vi "Global-IP_UI.vi"() -> ()   [LabVIEW 2021]
uses:
  IP_Cellular Tech Type def.ctl
  IP_Network_Type def.ctl
  IP_Type-Tydedef.ctl
panel:
  in  "IP_UI":T4(array[cluster])
  in  "IP_UI_Boolean":bool[](array[boolean])=[FALSE, FALSE, FALSE]
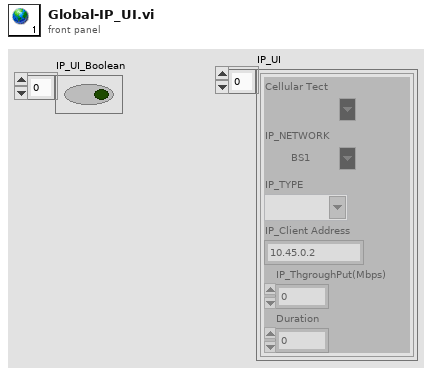
[diagram p1: front panel]
types:
  T1 = typedef "IP_Cellular Tech Type def.ctl" = string
  T2 = typedef "IP_Network_Type def.ctl" = string
  T3 = typedef "IP_Type-Tydedef.ctl" = string
  T4 = cluster{"Cellular Tect":T1, "IP_NETWORK":T2, "IP_TYPE":T3, "IP_Client Address":string, "IP_ThgroughPut(Mbps)":i32, "Duration":i32}[]
diagram:
